vi "Nominal Client.Async.vi"(10 "Parameters":variant, 11 "Process":refnum<class "Process.lvclass">) -> ()   [LabVIEW 2024, in "Nominal Client Engine.lvlib"]
uses:
  Nominal Client Engine.lvlib
  <vilib>/NI/NIVS Inline Async API/_VS Inline Async API/Process/Process.lvclass
  <vilib>/NI/NIVS Inline Async API/_VS Inline Async API/Process/Process.lvclass/Process.ctl
  Shared/Compiled.Settings.ctl
  Streaming Specification.ctl
  Group Buffer Data.ctl
  Property Specification.ctl
  <vilib>/NI/NIVS Inline Async API/_Data Access Engine/Access Type Classes/Read/Read.lvclass/Read.ctl
  <vilib>/NI/NIVS Inline Async API/_Data Access Engine/Data Access Engine/Methods/Read.Data.vi
  <vilib>/NI/NIVS Inline Async API/_VS Inline Async API/Process/Data Member Access/Read Data Access.vi
  <vilib>/NI/NIVS Inline Async API/_VS Inline Async API/Error Handling Process/SubVIs/Error.ConvertArray.vi
  <vilib>/NI/NIVS Inline Async API/_Data Access Engine/Access Type Classes/Read/Read.ProcessData.vi
  <vilib>/NI/NIVS Inline Async API/_Data Access Engine/Data Access Engine/Methods/Read.Lookup.vi
  <vilib>/NI/NIVS Inline Async API/_Data Access Engine/Data Access Engine/Data Access Engine.lvclass
  Shared/Nominal Client Shared.lvlib
  LabVIEW Client/nominal labview client.lvlib
panel:
  out "Response body":string
  out "Data Source RID":string
  out "transposed array":dbl[][](array[numeric])
  out "Timeout?":bool
  out "# elements in queue":i32
  out "overflow?":bool
  in  "milliseconds to wait":u32=10
  out "data":T1(array[cluster])
  out "loop period":dbl format="%#_10p"
  out "Streaming spec.Channels":string[](array[string])
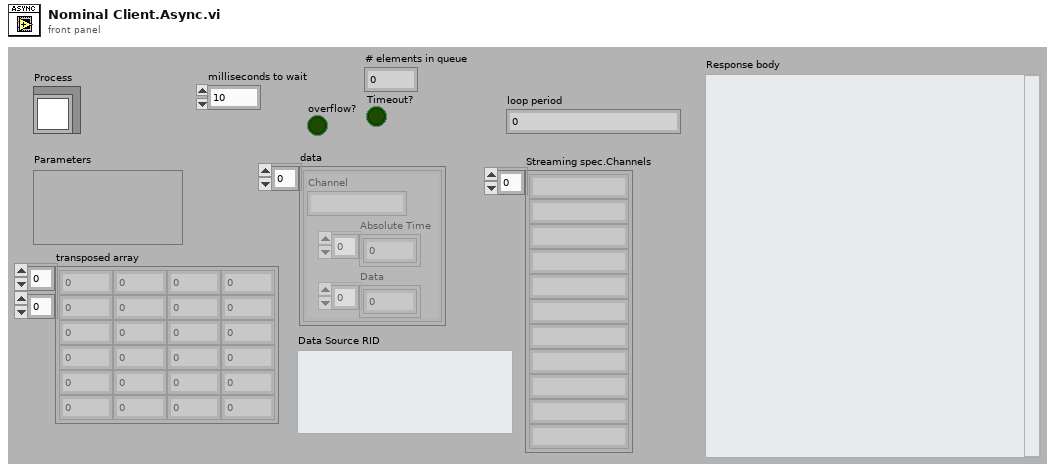
[diagram p1: front panel]
types:
  T1 = cluster{"Channel":string, "Absolute Time":dbl[], "Data":dbl[]}[]
  T2 = typedef "Nominal Client Shared.lvlib/Compiled.Settings.ctl" = cluster{"Name":string, "Async Init Timeout":u16, "api key":string, "datasource connection name":string, "create new datasource":bool}
  T3 = typedef "Nominal Client Engine.lvlib/Streaming Specification.ctl" = cluster{"Name":string, "Channels":string[], "Description":string, "Buffer Data":T4, "Channel Properties":cluster{"Array":T5[]}[], "dt":dbl}
  T4 = typedef "Nominal Client Engine.lvlib/Group Buffer Data.ctl" = cluster{"Last":i32, "Start":i32, "Length":i32, "Channel Count":i32, "Data":dbl[][], "Last Trigger":bool}
  T5 = typedef "Nominal Client Engine.lvlib/Property Specification.ctl" = cluster{"Name":string, "Value":variant}
  T6 = cluster{"Compiled.Settings":T2, "Streaming spec":T3}
  T7 = typedef "Data Access Engine.lvlib/Data Access Engine.lvclass/Read.DVR.ctl" = refnum<data-value>
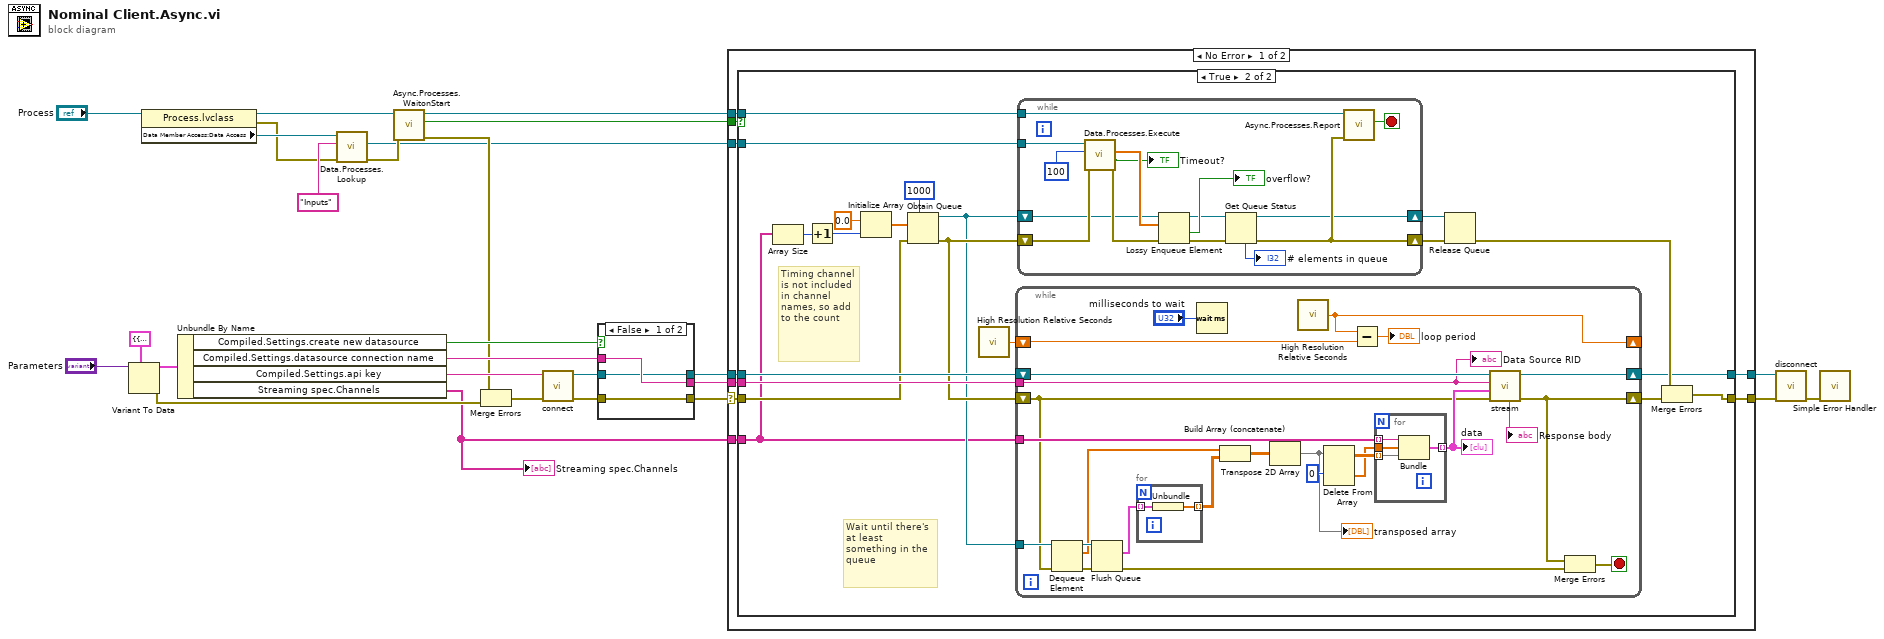
[diagram p0: block diagram]
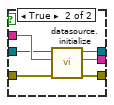
[diagram p2: hidden frame]
diagram:
  n1 = Variant To Data(type=T6 {"Compiled.Settings"={"Name"="", "Async Init Timeout"=0, "api key"="", "datasource connection name"="", "create new datasource"=FALSE}, "Streaming spec"={"Name"="", "Channels"=[], "Description"="", "Buffer Data"={"Last"=0, "Start"=0, "Length"=0, "Channel Count"=0, "Data"=[], "Last Trigger"=FALSE}, "Channel Properties"=[], "dt"=0.0}} ("cluster"), Variant="Parameters") -> (data=w21:T6, error out=w4:errorcluster)  [unwired: 1 in]
  n2 = property class="Process.lvclass"(reference="Process") -> (reference out=w22:refnum<class "Process.lvclass">, error out=w19:errorcluster, "Data Member Access:Data Access"=w20:refnum<class "Data Access Engine.lvclass">)  [unwired: 1 in]
  n3 = Unbundle By Name(w21) -> ("Compiled.Settings.create new datasource"=w6:bool, "Compiled.Settings.datasource connection name"=w16:string, "Compiled.Settings.api key"=w17:string, "Streaming spec.Channels"=w1:string[])
  "Streaming spec.Channels" <- w1
  n4 = call-poly <vilib>:"Data.Processes.Lookup.vi"("error in (no error)"=w19, "Name"="Inputs", "Data Access API in"=w20) -> ("error out"=w23:errorcluster, "Ref"=w2:T7)  [unwired: 5 in, 2 out]
  n5 = call <vilib>:"Async.Processes.WaitonStart.vi"("error in (no error)"=w23, "Process"=w22) -> ("error out"=w5:errorcluster, "Execute"=w25:bool, "Process out"=w7:refnum<class "Process.lvclass">)  [unwired: 7 in]
  n6 = Merge Errors(w5, w4) -> (w3:errorcluster)
  n7 = call "connect.vi"("error in"=w3, "API Token"=w17) -> ("error out"=w10:errorcluster, "Nominal Client"=w15:refnum<class "Nominal Client.lvclass">)  [unwired: 8 in]
  n8 = case shown="False" w6 {
    tunnel: w16 -> [w30 w36]
    tunnel: w15 -> [w29 w35]
    tunnel: [w29 w34] -> w14
    tunnel: [w30 w33] -> w13
    tunnel: w10 -> [w28 w32]
    tunnel: [w28 w31] -> w9
    frame False {
    }
    frame True {
      n9 = call "datasource.initialize.vi"("error in"=w32, "Datasource Name"=w36, "Nominal Client in"=w35) -> ("error out"=w31:errorcluster, "datasource rid"=w33:string, "Nominal Client out"=w34:refnum<class "Nominal Client.lvclass">)  [unwired: 6 in]
    }
  }
  n10 = case shown="No Error" w9 {
    selector: w9 -> [w44 w114]
    tunnel: w25 -> [w45 _]
    tunnel: w14 -> [w43 w115]
    tunnel: w13 -> [w42 _]
    tunnel: [w41 w115] -> w12
    tunnel: [w40 w114] -> w11
    tunnel: w2 -> [w39 _]
    tunnel: w7 -> [w38 _]
    tunnel: w1 -> [w37 _]
    frame No Error {
      n11 = case shown="True" w45 {
        tunnel: w44 -> [w46 w58]
        tunnel: w43 -> [w47 w66]
        tunnel: w42 -> [_ w65]
        tunnel: [w47 w51] -> w41
        tunnel: [w46 w53] -> w40
        tunnel: w39 -> [_ w64]
        tunnel: w38 -> [_ w63]
        tunnel: w37 -> [_ w48]
        frame False {
        }
        frame True {
          # "Wait until there's at least something in the queue"
          # "Timing channel is not included in channel names, so add to the count"
          n12 = Array Size(array=w48) -> (size(s)=w50:i32)
          n13 = Increment(x=w50) -> (x+1=w49:i32)
          n14 = Initialize Array(0.0 ("Channel Data Reference"), w49) -> (w61:dbl[])
          n15 = Obtain Queue(max queue size (-1, unlimited)=1000, element data type=w61, error in (no error)=w58) -> (queue out=w52:refnum<queue>, error out=w56:errorcluster)  [unwired: 2 in, 1 out]
          n16 = call <vilib>:"High Resolution Relative Seconds.vi"() -> ("relative seconds"=w67:dbl)
          n17 = while {
            shift-right: [w105] -> _
            shift-left: w67 -> [w106]
            tunnel: w65 -> [w91]
            tunnel: w48 -> [w100]
            tunnel: w52 -> [w90]
            shift-right: [w103] -> w51
            shift-left: w66 -> [w104]
            shift-right: [w96] -> w54
            shift-left: w56 -> [w87]
            stop <- w94 stop-if-true
            n18 = Dequeue Element(queue=w90, error in (no error)=w87) -> (queue out=w88:refnum<queue>, element=w85:dbl[], error out=w89:errorcluster)  [unwired: 1 in, 1 out]
            n19 = Flush Queue(queue=w88, error in (no error)=w89) -> (remaining elements=w97:cluster{dbl[]}[], error out=w95:errorcluster)  [unwired: 1 out]
            n20 = for {
              tunnel: w97 -> [w109] mode=indexing
              tunnel: [w108] -> w86 mode=indexing
              n21 = Unbundle(w109) -> (w108:dbl[])
            }
            n22 = Wait (ms)(milliseconds to wait="milliseconds to wait") -> ()  [unwired: 1 out]
            n23 = Build Array (concatenate)(w85, w86) -> (w84:dbl[][])
            n24 = Transpose 2D Array(2D array=w84) -> (transposed array=w92:dbl[][])
            "transposed array" <- w92
            n25 = call <vilib>:"High Resolution Relative Seconds.vi"() -> ("relative seconds"=w105:dbl)
            n26 = Delete From Array(array=w92, index (row)=0) -> (deleted portion=w99:dbl[], array with subset deleted=w101:dbl[][])  [unwired: 2 in]
            n27 = Subtract(x=w105, y=w106) -> (x-y=→"loop period":dbl)
            n28 = for {
              tunnel: w100 -> [w113] mode=indexing
              tunnel: w101 -> [w111] mode=indexing
              tunnel: w99 -> [w112]
              tunnel: [w110] -> w93 mode=indexing
              n29 = Bundle("String"=w113, w112, w111) -> (w110:cluster{"String":string, dbl[], dbl[]})  [unwired: 1 in]
            }
            "data" <- w93
            n30 = call "stream.vi"("error in"=w87, "Data"=w93, "Data Source RID"=w91, "Nominal Client in"=w104) -> ("error out"=w96:errorcluster, "Nominal Client out"=w103:refnum<class "Nominal Client.lvclass">, "Response body"=→"Response body":string)  [unwired: 5 in]
            n31 = Merge Errors(w96, w95) -> (w94:errorcluster)
            "Data Source RID" <- w91
          }
          n32 = while {
            tunnel: w64 -> [w82]
            tunnel: w63 -> [w80]
            shift-right: [w69] -> w62
            shift-left: w52 -> [w68]
            shift-right: [w70] -> w57
            shift-left: w56 -> [w76]
            stop <- w79 stop-if-true
            n33 = call-poly <vilib>:"Data.Processes.Execute.vi"("error in (no error)"=w76, "timeout ms"=100, "Ref"=w82) -> ("error out"=w75:errorcluster, "Timeout?"=→"Timeout?":bool, "Values"=w78:dbl[])  [unwired: 6 in]
            n34 = Lossy Enqueue Element(queue=w68, element=w78, error in (no error)=w75) -> (queue out=w74:refnum<queue>, overflow?=→"overflow?":bool, error out=w73:errorcluster)  [unwired: 1 out]
            n35 = Get Queue Status(queue=w74, error in (no error)=w73) -> (queue out=w69:refnum<queue>, error out=w70:errorcluster, # elements in queue=→"# elements in queue":i32)  [unwired: 1 in, 5 out]
            n36 = call <vilib>:"Async.Processes.Report.vi"("Error"=w70, "Process in"=w80) -> ("Stop"=w79:bool)  [unwired: 8 in, 1 out]
          }
          n37 = Release Queue(queue=w62, error in (no error)=w57) -> (error out=w55:errorcluster)  [unwired: 1 in, 2 out]
          n38 = Merge Errors(w55, w54) -> (w53:errorcluster)
        }
      }
    }
    frame Error {
    }
  }
  n39 = call "disconnect.vi"("error in"=w11, "Nominal Client"=w12) -> ("error out"=w8:errorcluster)  [unwired: 9 in]
  n40 = call <vilib>:"Simple Error Handler.vi"("error in (no error)"=w8) -> ()  [unwired: 4 in, 5 out]
